vi "Byte Buffer.Write (1D I16).vi"(7 "byte order (big-endian)":T1(ring), 8 "error in (no error)":errorcluster, 9 "values":i16[](array[numeric]), 10 "buffer offset":i32, 11 "buffer in":string) -> (0 "error out":errorcluster, 3 "buffer out":string)   [LabVIEW 2016, in "VeriStand Data.lvlib"]
uses:
  VeriStand Data.lvlib
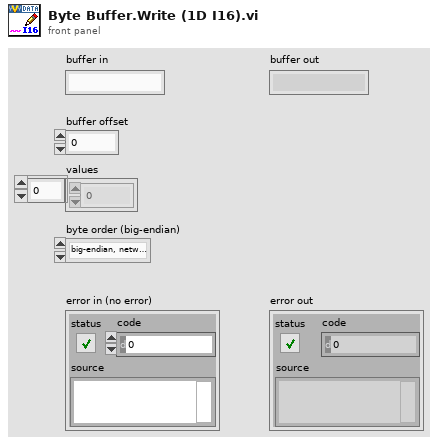
[diagram p1: front panel]
types:
  T1 = enum16{"big-endian, network order", "native, host order", "little-endian"}
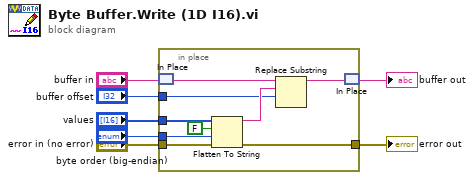
[diagram p0: block diagram]
diagram:
  n1 = in-place {
    in-place-border: "values" -> [w15]
    in-place-border: "buffer offset" -> [w12]
    in-place-border: "byte order (big-endian)" -> [w10]
    in-place-border: [w9] -> w2
    in-place-border: "error in (no error)" -> [w8]
    n2 = in-place-match #1("buffer in") -> (w16:string)
    n3 = Flatten To String(anything=w15, prepend array or string size? (T)=FALSE, byte order (0:big-endian, network order)=w10, error in (no error)=w8) -> (data string=w13:string, error out=w9:errorcluster)  [unwired: 1 out]
    n4 = Replace Substring(3:w12, 4:w13, 5:w16) -> (1:w11:string)  [unwired: 1 in, 1 out]
    n5 = in-place-match #1(w11) -> (→"buffer out":string)
  }
  "error out" <- w2
